vi "VI dependent on missing VI.vi"   [LabVIEW 2023]
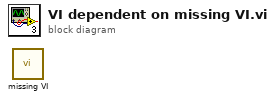
[diagram p0: block diagram]
diagram:
  n1 = call "missing VI.vi"() -> ()  [unwired: 12 in]
